vi "Write Read Loop with Config.vi"() -> (0 "error out":errorcluster)   [LabVIEW 2019]
panel:
  in  "Config Values":dbl[](array[numeric])=[10.0, 0.0] format="%.2f"
  in  "Config Names":string[](array[string])=["AIN0_RANGE", "AIN0_RESOLUTION_INDEX"]
  out "Iteration":u32
  in  "stop":bool
  in  "Interval [ms]":i32=500
  in  "Read Names":string[](array[string])=["AIN0", "FIO2"]
  in  "Write Values":dbl[](array[numeric])=[2.34, 1.0] format="%.2f"
  out "Error String":string
  out "ConnectionType Out":i32
  out "DeviceType Out":i32
  in  "Identifier":string="LJM_idANY"
  in  "ConnectionType":string="LJM_ctANY"
  in  "DeviceType":string="LJM_dtANY"
  out "Read Values":dbl[](array[numeric]) format="%.6f"
  in  "Write Names":string[](array[string])=["DAC0", "FIO1"]
  # "This is perhaps the most common program structure used, and a copy of this VI can be the starting point for many users.\n\nPerforms an initial call to eWriteNames to write configuration values, and then calls eReadNames & eWriteNames repeatedly in a loop.\n\nFor documentation on register names to use, see the T-series Datasheet or the Modbus Map.\n\nSome more advanced program structure examples can be found in \\Examples\\More\\Misc."
  # "All controls can be changed while running except the Open\nparameters and Config parameters.  You must stop the program\nto change these.\n\nTo remove an element, right-click on it, select\nData Operations => Remove Element.\n\nTo empty an array, right-click near the edge, select\nData Operations => Empty Array.\n\nOther useful operations:  From the Operate menu are \"Make Current\nValues Default\" and \"Reinitialize To Default\" (source only ... does\nnot work with exe)."
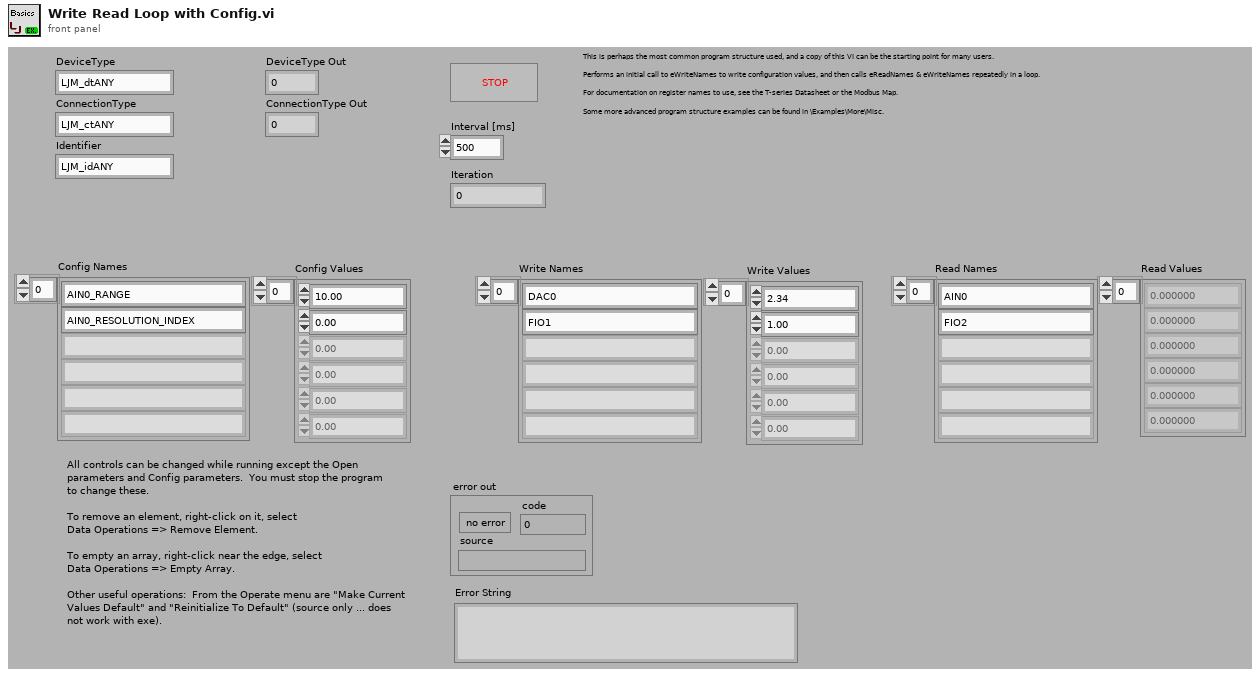
[diagram p1: front panel]
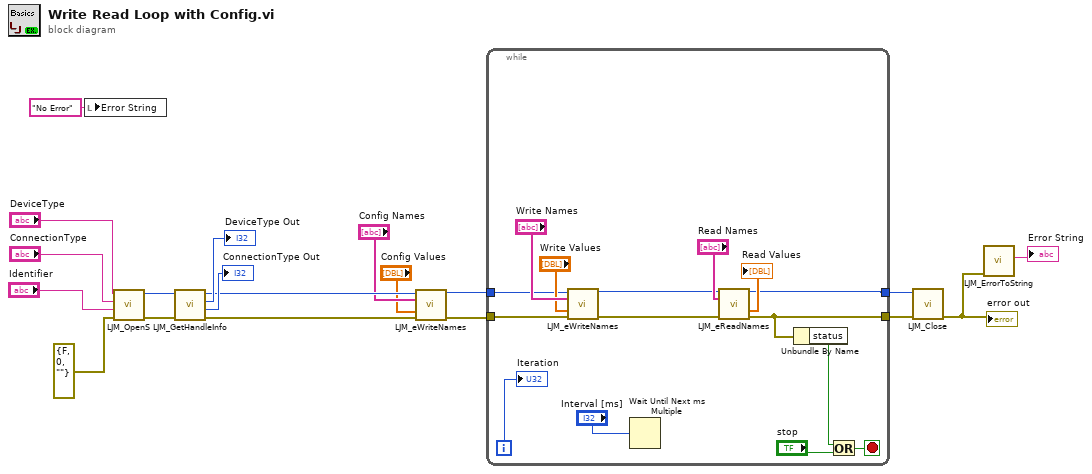
[diagram p0: block diagram]
diagram:
  n1 = local write "Error String"("No Error" ("Error String")) -> ()
  n2 = call "LJM_OpenS.vi"("error in"=errorcluster {"status"=FALSE, "code"=0, "source"=""} ("error in (no error)"), "Identifier"="Identifier", "ConnectionType"="ConnectionType", "DeviceType"="DeviceType") -> ("error out"=w18:errorcluster, "Handle"=w17:i32)  [unwired: 6 in]
  n3 = call "LJM_GetHandleInfo.vi"("error in"=w18, "Handle In"=w17) -> ("error out"=w4:errorcluster, "ConnectionType"=→"ConnectionType Out":i32, "DeviceType"=→"DeviceType Out":i32, "Handle Out"=w5:i32)  [unwired: 2 in, 4 out]
  n4 = call "LJM_eWriteNames.vi"("Handle In"=w5, "aNames"="Config Names", "aValuesIn"="Config Values", "error in"=w4) -> ("Handle Out"=w7:i32, "error out"=w6:errorcluster)  [unwired: 9 in, 1 out]
  n5 = while {
    tunnel: w6 -> [w23]
    tunnel: [w25] -> w9
    tunnel: w7 -> [w22]
    tunnel: [w20] -> w8
    i -> [w26]
    stop <- w32 stop-if-true
    n6 = call "LJM_eWriteNames.vi"("Handle In"=w22, "aNames"="Write Names", "aValuesIn"="Write Values", "error in"=w23) -> ("Handle Out"=w21:i32, "error out"=w24:errorcluster)  [unwired: 9 in, 1 out]
    n7 = Wait Until Next ms Multiple(millisecond multiple="Interval [ms]") -> ()  [unwired: 1 out]
    n8 = call "LJM_eReadNames.vi"("Handle In"=w21, "aNames"="Read Names", "error in"=w24) -> ("Handle Out"=w20:i32, "aValuesOut"=→"Read Values":dbl[], "error out"=w25:errorcluster)  [unwired: 9 in, 1 out]
    n9 = Unbundle By Name(w25) -> ("status"=w31:bool)
    n10 = Or(x=w31, y="stop") -> (x .or. y?=w32:bool)
    "Iteration" <- w26
  }
  n11 = call "LJM_Close.vi"("error in"=w9, "Handle"=w8) -> ("error out"=w11:errorcluster)  [unwired: 9 in]
  "error out" <- w11
  n12 = call "LJM_ErrorToString.vi"("error in"=w11) -> ("String"=→"Error String":string)  [unwired: 10 in]
